vi "controllerMain.vi"(8 "error in (no error)":errorcluster, 10 "UserEvents in":refnum<class "UserEvents.lvclass">, 11 "Controller in":refnum<class "Controller.lvclass">) -> (0 "error out":errorcluster, 3 "Controller out":refnum<class "Controller.lvclass">)   [LabVIEW 2013, in "Controller.lvclass"]
uses:
  Controller.lvclass
  UserEvents/UserEvents.lvclass
  StateFactory/StateFactory.lvclass
  Typedefs/StateSelector.ctl
  Model/Model/Model/Model.lvclass
  Context/Context.lvclass
  CommandFactory/CommandFactory.lvclass
  Model/SDAFactory/SDAFactory.lvclass
  <userlib>/Common/SerialProtocols/SerialProtocolFactory/SerialProtocolFactory/SerialProtocolFactory.lvclass
  <userlib>/Common/SerialProtocols/SerialCommunicator/SerialCommunicator.lvclass
  Model/ILCTC/ILCTC.lvclass
  Model/ILCSim1TC/ILCSim1TC.lvclass
  <userlib>/Common/SerialProtocols/SerialCommunicator/SerialCommunicator.lvclass/SerialCommunicator.ctl
  <userlib>/Common/ILC/ILC/ILC.lvclass/ILC.ctl
  <vilib>/Platform/TimedLoop/XDataNode/timing_clust.ctl
  <vilib>/Platform/TimedLoop/XDataNode/nitl_modes.ctl
  <vilib>/Platform/TimedLoop/XDataNode/wakeup.ctl
  UserEvents/UserEvents.lvclass/UserEvents.ctl
  Model/Model/Model/Model.lvclass/Model.ctl
  Context/Context.lvclass/Context.ctl
  Typedefs/CommandSelector.ctl
  Command/Command.lvclass
  <vilib>/platform/TimedLoop/XDataNode/XDataNode.xnode
  <vilib>/Platform/TimedLoop/XDataNode/XDNodeRunTimeDep.lvlib
  <userlib>/Common/ILC/ILC/ILC.lvclass
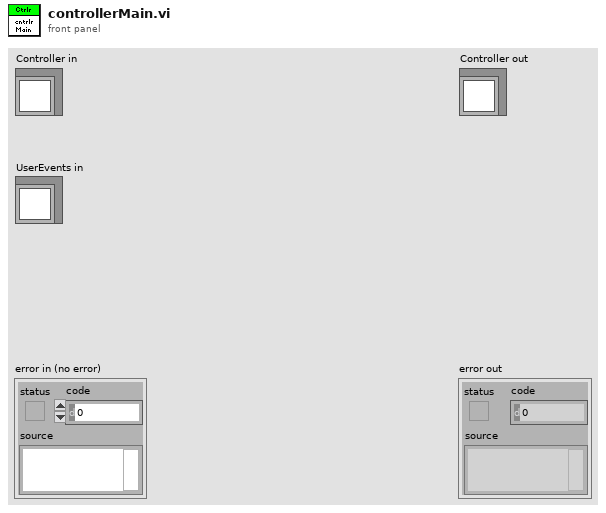
[diagram p1: front panel]
types:
  T1 = typedef "StateSelector.ctl" = enum16{"DataOnDemandState", "DataStreamingState", "FaultState", "OffState", "StandbyState"}
  T2 = typedef "PubDataEvents.ctl" = cluster{"State":refnum<user-event>, "ErrorCode":refnum<user-event>, "OutputData":refnum<user-event>, "InputData":refnum<user-event>, "NeedUserOutputs":refnum<user-event>}
  T3 = typedef "SubDataEvents.ctl" = cluster{"Command":refnum<user-event>}
  T4 = typedef "XDNodeRunTimeDep.lvlib/timing_clust.ctl" = cluster{"Expected End [f-1]":u64, "Actual End [f-1]":u64, "Finished Late? [f-1]":bool, "Expected End [i-1]":u64, "Actual End [i-1]":u64, "Finished Late? [i-1]":bool, "Expected Start [i]":u64, "Actual Start [i]":u64, "Expected Start [f]":u64, "Actual Start [f]":u64, "Source Name":string, "Structure Name":string, "Period":i64, "Deadline":i64, "Offset":i64, "Start":i64, "Priority":i32, "Timeout":i32, "Mode":T5, "Wakeup Reason":T6, "Error":errorcluster, "Source Type":string, "Secondary Source Type":string, "Global End Time":u64, "Global Start Time":u64, "Frame Duration":u64, "Iteration Duration":u64, "Assigned CPU":i32, "I/O Scan Engine Mode":u32}
  T5 = typedef "XDNodeRunTimeDep.lvlib/nitl_modes.ctl" = enum32{"No Change", "Process missed periods, maintain original phase", "Discard missed periods, maintain original phase", "Process missed periods, ignore original phase", "Discard missed periods, ignore original phase"}
  T6 = typedef "XDNodeRunTimeDep.lvlib/wakeup.ctl" = enum32{"Normal", "Aborted", "Asynchronous wakeup", "Timing source error", "Timed loop error", "Timeout"}
  T7 = typedef "CommandSelector.ctl" = enum16{"ClearError", "Exit", "StandBy", "Start", "SwitchToOnDemandMode", "SwitchToStreamMode", "Update"}
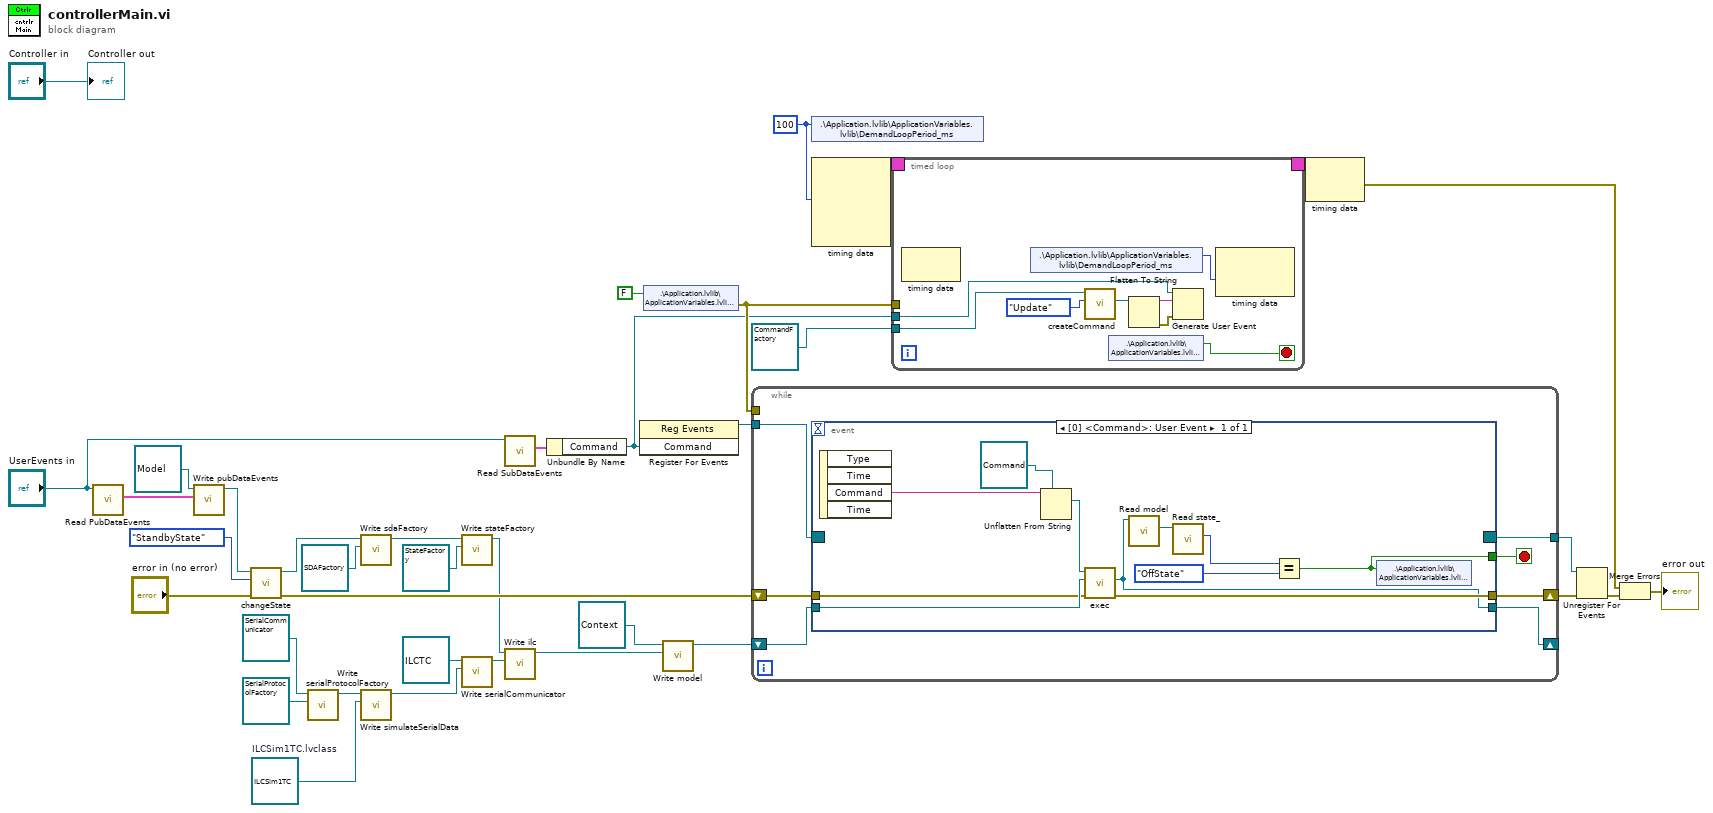
[diagram p0: block diagram]
diagram:
  w1 = refnum<class "ILCSim1TC.lvclass"> refnum  # ILCSim1TC.lvclass
  w10 = i64 100 ("Period")
  n1 = call "Read PubDataEvents.vi"("UserEvents in"="UserEvents in") -> ("PubDataEvents"=w15:T2)  [unwired: 9 in, 1 out]
  n2 = call "Write pubDataEvents.vi"("pubDataEvents"=w15, "Model in"=refnum<class "Model.lvclass"> refnum) -> ("Model out"=w18:refnum<class "Model.lvclass">)  [unwired: 9 in]
  n3 = call "changeState.vi"("error in (no error)"="error in (no error)", "State:"=StateSelector."StandbyState", "Model in"=w18) -> ("error out"=w20:errorcluster, "Model out"=w27:refnum<class "Model.lvclass">)  [unwired: 7 in]
  n4 = call <userlib>:"Write serialProtocolFactory.vi"("serialProtocolFactory"=refnum<class "SerialProtocolFactory.lvclass"> refnum ("SerialCommFactory.lvclass"), "SerialCommunicator in"=refnum<class "SerialCommunicator.lvclass"> refnum ("SerialProtocols.lvlib:SerialCommunicator.lvclass")) -> ("SerialCommunicator out"=w3:refnum<class "SerialCommunicator.lvclass">)  [unwired: 9 in]
  n5 = call "Write sdaFactory.vi"("sdaFactory"=refnum<class "SDAFactory.lvclass"> refnum ("SDAFactory.lvclass"), "Model in"=w27) -> ("Model out"=w26:refnum<class "Model.lvclass">)  [unwired: 9 in]
  n6 = call <userlib>:"Write simulateSerialData.vi"("simulateSerialData"=w1, "SerialCommunicator in"=w3) -> ("SerialCommunicator out"=w2:refnum<class "SerialCommunicator.lvclass">)  [unwired: 9 in]
  n7 = call "Write stateFactory.vi"("stateFactory"=refnum<class "StateFactory.lvclass"> refnum ("StateFactory.lvclass"), "Model in"=w26) -> ("Model out"=w5:refnum<class "Model.lvclass">)  [unwired: 9 in]
  n8 = call <userlib>:"Write serialCommunicator.vi"("serialCommunicator"=w2, "ILC in"=refnum<class "ILCTC.lvclass"> refnum ("ILCTC.lvclass")) -> ("ILC out"=w6:refnum<class "ILCTC.lvclass">)  [unwired: 9 in]
  n9 = call "Read SubDataEvents.vi"("UserEvents in"="UserEvents in") -> ("SubDataEvents"=w24:T3)  [unwired: 9 in, 1 out]
  n10 = call "Write ilc.vi"("ilc"=w6, "Model in"=w5) -> ("Model out"=w4:refnum<class "Model.lvclass">)  [unwired: 9 in]
  n11 = Unbundle By Name(w24) -> ("Command"=w12:refnum<user-event>)
  n12 = register-events(w12) -> (reference out=w23:refnum<event-registration>)  [unwired: 2 in, 1 out]
  n13 = shared-variable ".\\Application.lvlib\\ApplicationVariables.lvlib\\ExitIsTrue"(FALSE ("ExitIsTrue")) -> (error out=w28:errorcluster)  [unwired: 1 in]
  n14 = call "Write model.vi"("Model.lvclass"=w4, "Context in"=refnum<class "Context.lvclass"> refnum ("Context.lvclass")) -> ("Context out"=w34:refnum<class "Context.lvclass">)  [unwired: 9 in]
  n15 = while {
    shift-right: [w43] -> w21
    shift-left: w20 -> [w40]
    shift-right: [w42] -> _
    shift-left: w34 -> [w44]
    tunnel: w28 -> [_]
    tunnel: w23 -> [w39]
    tunnel: [w38] -> w22
    stop <- w41 stop-if-true
    n16 = event shown="[0] <Command>: User Event" {
      selector: w39 -> [_]
      dyn-events: [_] -> w38
      timeout: _ -> [_]
      tunnel: w44 -> [w53]
      tunnel: [w50] -> w43
      tunnel: [w49] -> w42
      tunnel: [w48] -> w41
      tunnel: w40 -> [w46]
      event User Event {
        n17 = event-data() -> ("Command"=w45:string)  [unwired: 1 in, 3 out]
        n18 = Unflatten From String(type=refnum<class "Command.lvclass"> refnum ("Command.lvclass"), binary string=w45) -> (value=w54:refnum<class "Command.lvclass">)  [unwired: 3 in, 2 out]
        n19 = call-dynamic "exec.vi"("error in (no error)"=w46, "context"=w53, "Command in"=w54) -> ("error out"=w50:errorcluster, "context 2"=w49:refnum<class "Context.lvclass">)  [unwired: 6 in, 1 out]
        n20 = call "Read model.vi"("Context in"=w49) -> ("Model.lvclass"=w52:refnum<class "Model.lvclass">)  [unwired: 9 in, 1 out]
        n21 = call "Read state_.vi"("Model in"=w52) -> ("state:"=w47:T1)  [unwired: 9 in, 1 out]
        n22 = Equal?(x=w47, y=StateSelector."OffState") -> (x = y?=w48:bool)
        n23 = shared-variable ".\\Application.lvlib\\ApplicationVariables.lvlib\\ExitIsTrue"(w48) -> ()  [unwired: 1 in, 1 out]
      }
    }
  }
  n24 = shared-variable ".\\Application.lvlib\\ApplicationVariables.lvlib\\DemandLoopPeriod_ms"(w10) -> ()  [unwired: 1 in, 1 out]
  n25 = node-c288(w10) -> (w30:T4)  [unwired: 3 in]
  n26 = timed-loop {
    timing: w30 -> [_]
    timing-out: [_] -> w29
    tunnel: refnum<class "CommandFactory.lvclass"> refnum ("CommandFactory.lvclass") -> [w62]
    tunnel: w28 -> [_]
    tunnel: w12 -> [w58]
    stop <- w60 stop-if-true
    n27 = node-c288() -> ()  [unwired: 1 in, 1 out]
    n28 = shared-variable ".\\Application.lvlib\\ApplicationVariables.lvlib\\DemandLoopPeriod_ms"() -> (w56:i64)  [unwired: 1 in, 1 out]
    n29 = call-dynamic "createCommand.vi"("Command"=CommandSelector."Update", "CommandFactory in"=w62) -> ("command"=w61:refnum<class "Command.lvclass">)  [unwired: 7 in, 2 out]
    n30 = shared-variable ".\\Application.lvlib\\ApplicationVariables.lvlib\\ExitIsTrue"() -> (w60:bool)  [unwired: 1 in, 1 out]
    n31 = Flatten To String(anything=w61) -> (data string=w57:string, error out=w59:errorcluster)  [unwired: 3 in, 1 out]
    n32 = Generate User Event(user event=w58, event data cluster=w57, error in=w59) -> ()  [unwired: 1 in, 2 out]
    n33 = node-c288(w56) -> ()  [unwired: 1 in, 1 out]
  }
  n34 = node-c288(w29) -> (w14:errorcluster)
  n35 = Unregister For Events(event registration refnum=w22, error in=w21) -> (error out=w13:errorcluster)
  n36 = Merge Errors(w14, w13) -> (→"error out":errorcluster)
  "Controller out" <- "Controller in"
